vi "Chroma 1905x Series Start and Get Data.vi"(0 "inst handle in":refnum<visa-resource-name>, 3 "error in":T1) -> (1 "Voltage":string, 4 "Judgement Overall":string, 5 "Current":string, 6 "inst handle out":refnum<visa-resource-name>, 8 "Judgement Last Test":string, 9 "error out":T1)   [LabVIEW 2025]
doc: "Contact Chroma\nTEL: +886-2-2298-3855 \nTEL: +886-3-397-5788 \nFAX: +886-2-2298-3596\nFAX: +886-3-327-4703 \nURL: http://www.chromaate.com \nE-mail: chroma@chroma.com.tw"
panel:
  out "number":dbl format="%.2f"
  out "Result":string
  # "Start and Get Data"
  # "Judgement\n120-121 Fail\n116   Pass\n115   Testing\n114   Cannot Test\n113   User Stop\n112   Stop\n17 - 55 Fail"
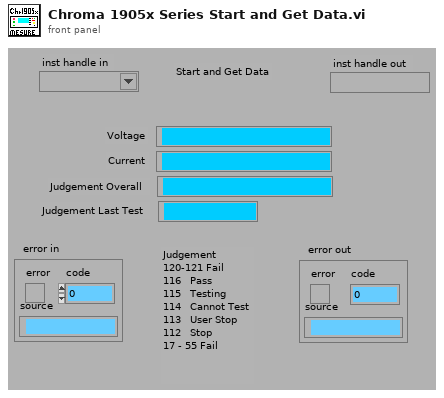
[diagram p1: front panel]
types:
  T1 = cluster{"error":bool, "code":i8, "source":string}
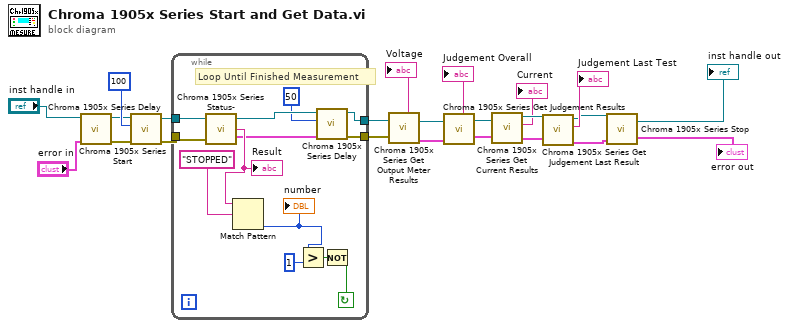
[diagram p0: block diagram]
diagram:
  n1 = call "Chroma 1905x Series Start.vi"("error in (no error)"="error in", "VISA resource name"="inst handle in") -> ("error out"=w2:errorcluster, "VISA resource name out"=w1:refnum<visa-resource-name>)  [unwired: 8 in]
  n2 = call "Chroma 1905x Series Delay.vi"("error in (no error)"=w2, "Time Delay [ms]"=u32 100 ("Time Delay S"), "VISA resource name"=w1) -> ("error out"=w22:errorcluster, "VISA resource name 2"=w21:refnum<visa-resource-name>)  [unwired: 7 in]
  n3 = while {
    tunnel: [w25] -> w19
    tunnel: [w27] -> w20
    tunnel: w22 -> [w35]
    tunnel: w21 -> [w36]
    stop <- w29 continue-if-true
    # "Loop Until Finished Measurement"
    n4 = call "Chroma 1905x Series Status-.vi"("error in"=w35, "inst handle in"=w36) -> ("error out"=w28:T1, "Status"=w33:string, "inst handle out"=w26:refnum<visa-resource-name>)  [unwired: 1 in]
    "Result" <- w33
    n5 = Match Pattern(string=w33, regular expression="STOPPED" ("format string")) -> (offset past match=w32:i32)  [unwired: 1 in, 3 out]
    "number" <- w32
    n6 = Greater?(x=w32, y=1) -> (0:w30:bool)
    n7 = call "Chroma 1905x Series Delay.vi"("error in (no error)"=w28, "Time Delay [ms]"=u32 50 ("Time Delay S"), "VISA resource name"=w26) -> ("error out"=w27:errorcluster, "VISA resource name 2"=w25:refnum<visa-resource-name>)  [unwired: 7 in]
    n8 = Not(x=w30) -> (.not. x?=w29:bool)
  }
  n9 = call "Chroma 1905x Series Get Output Meter Results.vi"("inst handle Out"=w19, "error in"=w20) -> ("inst handle in"=w18:refnum<visa-resource-name>, "Result"=→"Voltage":string, "error out"=w9:T1)  [unwired: 1 in]
  n10 = call "Chroma 1905x Series Get Judgement Results.vi"("inst handle Out"=w18, "error in"=w9) -> ("inst handle in"=w16:refnum<visa-resource-name>, "Result"=→"Judgement Overall":string, "error out"=w17:T1)  [unwired: 1 in]
  n11 = call "Chroma 1905x Series Get Current Results.vi"("inst handle Out"=w16, "error in"=w17) -> ("inst handle in"=w13:refnum<visa-resource-name>, "Result"=→"Current":string, "error out"=w12:T1)  [unwired: 1 in]
  n12 = call "Chroma 1905x Series Get Judgement Last Result.vi"("inst handle Out"=w13, "error in"=w12) -> ("inst handle in"=w8:refnum<visa-resource-name>, "Result"=→"Judgement Last Test":string, "error out"=w6:T1)  [unwired: 1 in]
  n13 = call "Chroma 1905x Series Stop.vi"("error in"=w6, "inst handle in"=w8) -> ("error out"=→"error out":T1, "inst handle out"=→"inst handle out":refnum<visa-resource-name>)  [unwired: 1 in]
